vi "CM_CalcVelocities.vi"(10 "Rotações":dbl[](array[numeric]), 11 "CM_data":T1[](array[typedef])) -> (3 "Velocidades":dbl[](array[numeric]))   [LabVIEW 2016]
uses:
  CM_data.ctl
  CM_SerialNumber.ctl
panel:
  out "equations":string[](array[string])
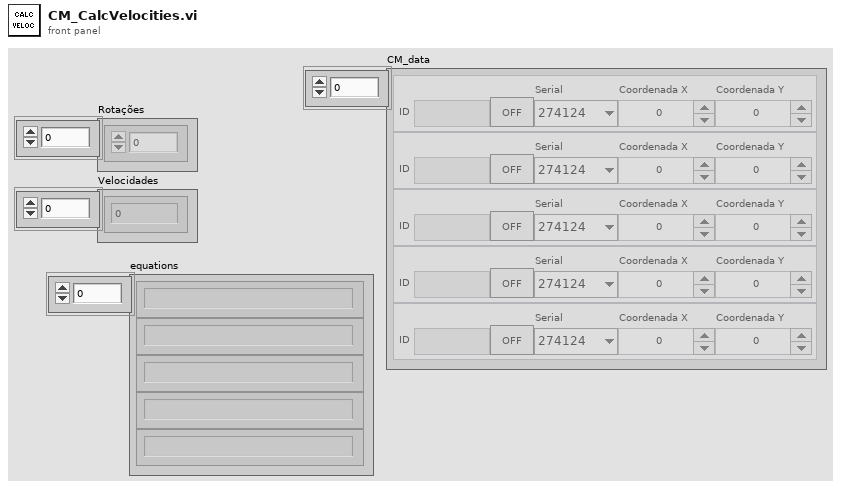
[diagram p1: front panel]
types:
  T1 = typedef "CM_data.ctl" = cluster{"Serial":T2, "Coordenada X":dbl, "Coordenada Y":dbl, "ID":string, "active":bool}
  T2 = typedef "CM_SerialNumber.ctl" = enum16{"274124", "274125", "274126", "274127", "274128"}
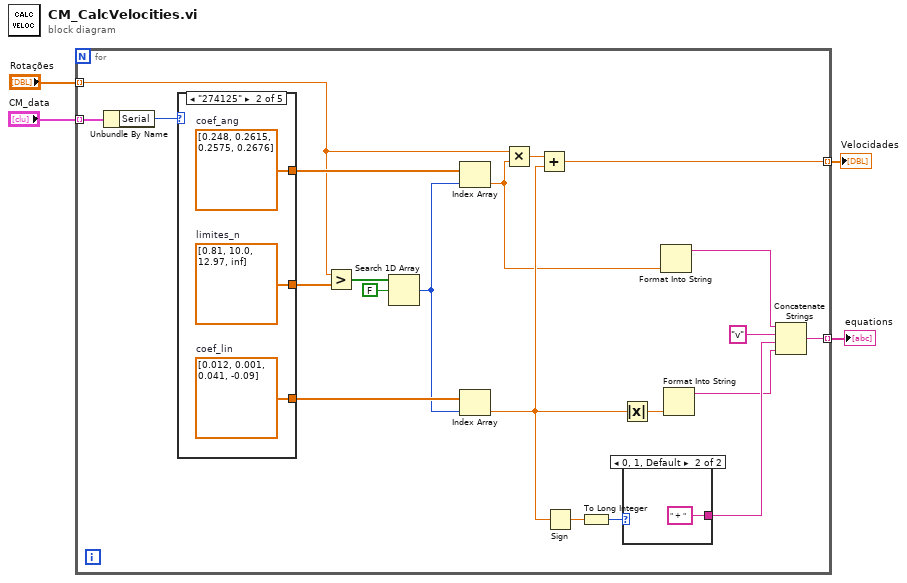
[diagram p0: block diagram]
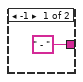
[diagram p2: hidden frame]
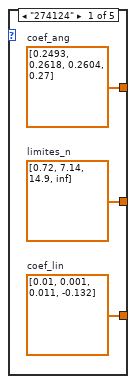
[diagram p3: hidden frame]
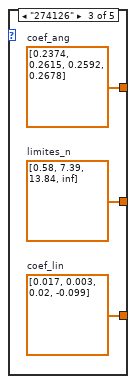
[diagram p4: hidden frame]
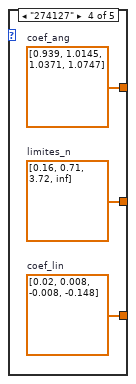
[diagram p5: hidden frame]
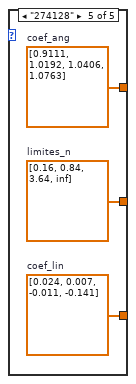
[diagram p6: hidden frame]
diagram:
  n1 = for {
    tunnel: "CM_data" -> [w9] mode=indexing
    tunnel: [w7] -> w2 mode=indexing
    tunnel: [w6] -> w3 mode=indexing
    tunnel: "Rotações" -> [w5] mode=indexing
    n2 = Unbundle By Name(w9) -> ("Serial"=w8:T2)
    n3 = case shown="\"274125\"" w8 {
      tunnel: [w29 w32 w35 w39 w41] -> w25
      tunnel: [w30 w33 w36 w38 w42] -> w22
      tunnel: [w28 w31 w34 w37 w40] -> w21
      frame "274124" {
        w28 = dbl[] [0.01, 0.001, 0.011, -0.132]  # coef_lin
        w30 = dbl[] [0.2493, 0.2618, 0.2604, 0.27]  # coef_ang
        w29 = dbl[] [0.72, 7.14, 14.9, inf]  # limites_n
      }
      frame "274125" {
        w31 = dbl[] [0.012, 0.001, 0.041, -0.09]  # coef_lin
        w33 = dbl[] [0.248, 0.2615, 0.2575, 0.2676]  # coef_ang
        w32 = dbl[] [0.81, 10.0, 12.97, inf]  # limites_n
      }
      frame "274126" {
        w34 = dbl[] [0.017, 0.003, 0.02, -0.099]  # coef_lin
        w36 = dbl[] [0.2374, 0.2615, 0.2592, 0.2678]  # coef_ang
        w35 = dbl[] [0.58, 7.39, 13.84, inf]  # limites_n
      }
      frame "274127" {
        w37 = dbl[] [0.02, 0.008, -0.008, -0.148]  # coef_lin
        w38 = dbl[] [0.939, 1.0145, 1.0371, 1.0747]  # coef_ang
        w39 = dbl[] [0.16, 0.71, 3.72, inf]  # limites_n
      }
      frame "274128" {
        w40 = dbl[] [0.024, 0.007, -0.011, -0.141]  # coef_lin
        w42 = dbl[] [0.9111, 1.0192, 1.0406, 1.0763]  # coef_ang
        w41 = dbl[] [0.16, 0.84, 3.64, inf]  # limites_n
      }
    }
    n4 = Greater?(x=w5, y=w25) -> (0:w24:bool[])
    n5 = Search 1D Array(1D array=w24, element=FALSE) -> (index of element=w10:i32)  [unwired: 1 in]
    n6 = Index Array(array=w22, index=w10) -> (element=w11:dbl)
    n7 = Index Array(array=w21, index=w10) -> (element=w19:dbl)
    n8 = Multiply(x=w5, y=w11) -> (x*y=w20:dbl)
    n9 = Add(x=w20, y=w19) -> (x+y=w7:dbl)
    n10 = Sign(1:w19) -> (0:w17:dbl)
    n11 = To Long Integer(number=w17) -> (32bit integer=w16:i32)
    n12 = Absolute Value(x=w19) -> (abs(x)=w18:dbl)
    n13 = case shown="0, 1, Default" w16 {
      tunnel: [" - " " + "] -> w13
      frame -1 {
      }
      frame 0, 1, Default {
      }
    }
    n14 = Format Into String(w11) -> (resulting string=w15:string)  [unwired: 3 in, 1 out]
    n15 = Format Into String(w18) -> (resulting string=w12:string)  [unwired: 3 in, 1 out]
    n16 = Concatenate Strings(w15, "v" ("string"), w13, w12) -> (w6:string)
  }
  "Velocidades" <- w2
  "equations" <- w3
